vi "Copy&FillNumber.vi"(8 "Length":i32=10, 9 "Level In":dbl format="%#_13g", 11 "Array In":dbl[](array[numeric])) -> (3 "Array Out":dbl[](array[numeric]))   [LabVIEW 2017]
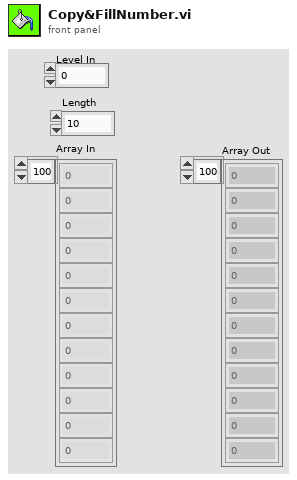
[diagram p1: front panel]
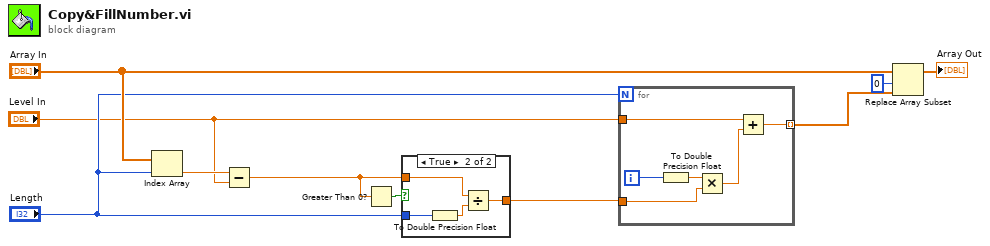
[diagram p0: block diagram]
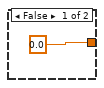
[diagram p2: hidden frame]
diagram:
  n1 = Index Array(array="Array In", index="Length") -> (element=w3:dbl)
  n2 = Subtract(x=w3, y="Level In") -> (x-y=w1:dbl)
  n3 = Greater Than 0?(x=w1) -> (x > 0?=w10:bool)
  n4 = case shown="True" w10 {
    tunnel: [0.0 w12] -> w4
    tunnel: w1 -> [_ w14]
    tunnel: "Length" -> [_ w13]
    frame False {
    }
    frame True {
      n5 = To Double Precision Float(number=w13) -> (double precision float=w15:dbl)
      n6 = Divide(x=w14, y=w15) -> (x/y=w12:dbl)
    }
  }
  n7 = for {
    N: "Length" -> [_]
    tunnel: w4 -> [w19]
    tunnel: [w17] -> w6 mode=indexing
    tunnel: "Level In" -> [w16]
    i -> [w20]
    n8 = To Double Precision Float(number=w20) -> (double precision float=w21:dbl)
    n9 = Multiply(x=w21, y=w19) -> (x*y=w18:dbl)
    n10 = Add(x=w16, y=w18) -> (x+y=w17:dbl)
  }
  n11 = Replace Array Subset(array="Array In", new element=w6, index=0) -> (→"Array Out":dbl[])
